vi "Peek.vi"(8 "error in (no error)":errorcluster, 11 "JSON Lexer in":refnum<class "JSON Lexer.lvclass">) -> (0 "error out":errorcluster, 1 "EOF":bool, 2 "Rune":string, 3 "JSON Lexer out":refnum<class "JSON Lexer.lvclass">)   [LabVIEW 2019, in "JKI JSON Serialization.lvlib" / "JSON Lexer.lvclass"]
doc: "JKI JSON 1.1.10.37\nTomi Maila - JKI\nCopyright (c) 2017, JKI"
uses:
  JSON Lexer.lvclass
  JSON Lexer.lvclass/JSON Lexer.ctl
  Unicode/UTF-8 String/UTF-8 String.lvclass/UTF-8 String.ctl
  Unicode/UTF-8 String/Index Rune as UTF-8 Substring.vi
  Unicode/UTF-8 String/Next Rune As UTF-8 Substring.vi
  Unicode/UTF-8 String/Bytes In Rune.vi
  <vilib>/Utility/error.llb/Error Cluster From Error Code.vi
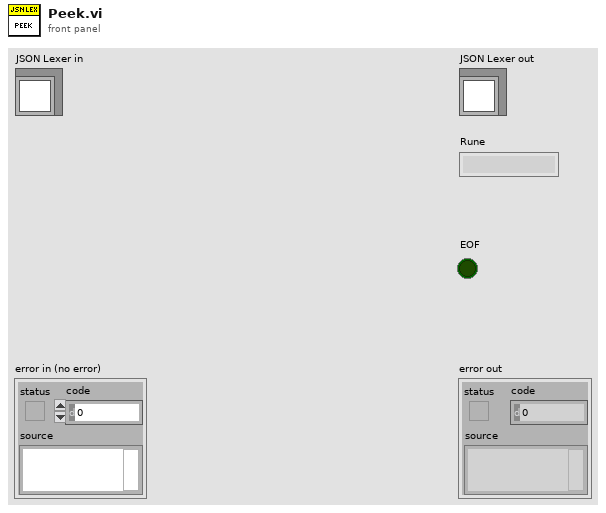
[diagram p1: front panel]
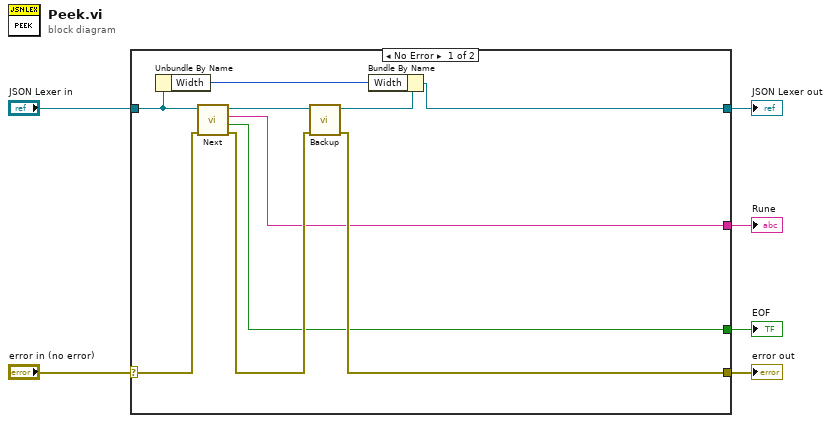
[diagram p0: block diagram]
diagram:
  n1 = case shown="No Error" "error in (no error)" {
    selector: "error in (no error)" -> [w16 w18]
    tunnel: [w13 w18] -> w5
    tunnel: [w8 w17] -> w3
    tunnel: "JSON Lexer in" -> [w10 w17]
    tunnel: [w12 _] -> w2
    tunnel: [w11 _] -> w1
    frame No Error {
      n2 = Unbundle By Name(w10) -> ("Width"=w7:i32)
      n3 = call "Next.vi"("error in (no error)"=w16, "JSON Lexer in"=w10) -> ("error out"=w14:errorcluster, "EOF"=w11:bool, "Rune"=w12:string, "JSON Lexer out"=w15:refnum<class "JSON Lexer.lvclass">)  [unwired: 6 in]
      n4 = call "Backup.vi"("error in (no error)"=w14, "JSON Lexer in"=w15) -> ("error out"=w13:errorcluster, "JSON Lexer out"=w9:refnum<class "JSON Lexer.lvclass">)  [unwired: 8 in]
      n5 = Bundle By Name(cluster=w9, "Width"=w7) -> (w8:refnum<class "JSON Lexer.lvclass">)
    }
    frame Error {
    }
  }
  "error out" <- w5
  "JSON Lexer out" <- w3
  "Rune" <- w2
  "EOF" <- w1
